vi "Make path.vi"(8 "error in (no error)":errorcluster, 10 "File type":T1, 11 "Tomo in":refnum<class "Tomo.lvclass">) -> (0 "error out":errorcluster, 2 "path":path, 3 "Tomo out":refnum<class "Tomo.lvclass">)   [LabVIEW 2012, in "Tomo.lvclass"]
uses:
  Tomo.lvclass
  file type.ctl
  Tomo.lvclass/Tomo.ctl
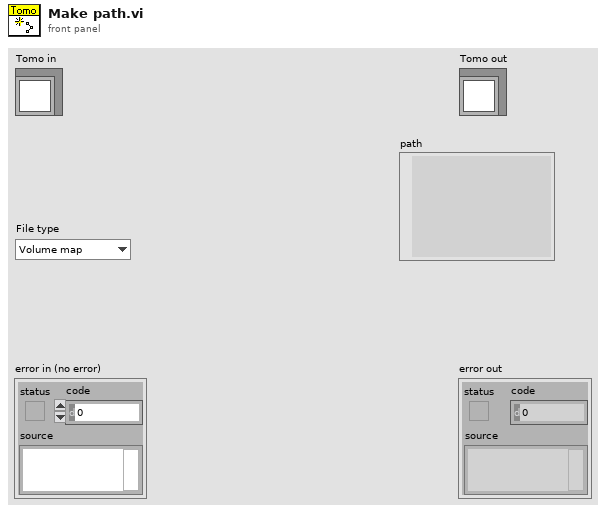
[diagram p1: front panel]
types:
  T1 = typedef "Tomo.lvclass/file type.ctl" = enum16{"Volume map", "Completed stacks"}
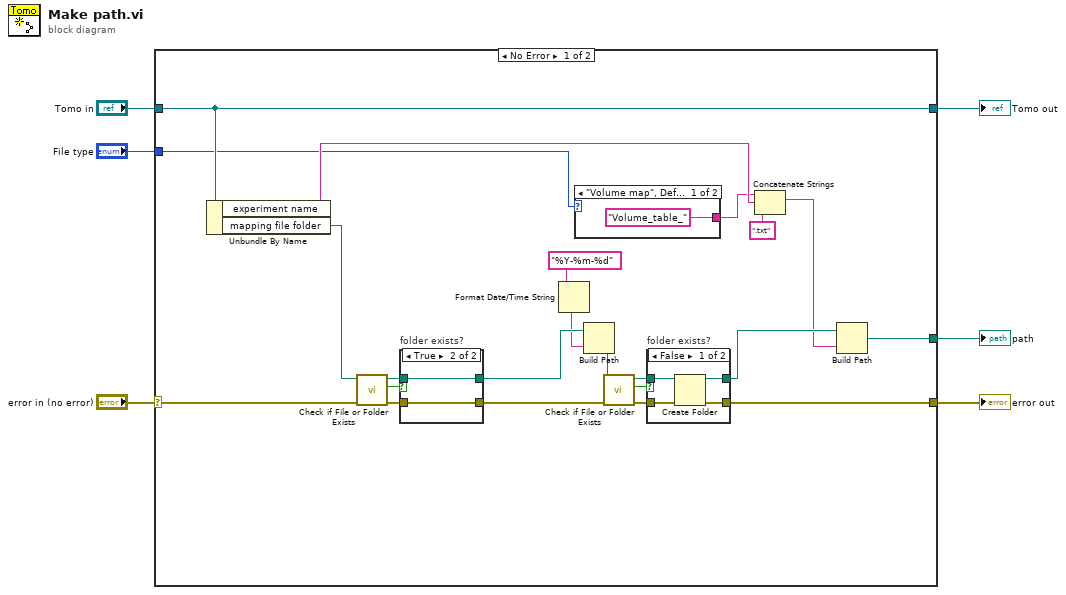
[diagram p0: block diagram]
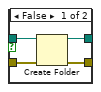
[diagram p3: hidden frame]
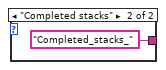
[diagram p4: hidden frame]
diagram:
  n1 = case shown="No Error" "error in (no error)" {
    selector: "error in (no error)" -> [w11 w44]
    tunnel: [w10 w44] -> w5
    tunnel: [w26 w43] -> w3
    tunnel: "Tomo in" -> [w26 w43]
    tunnel: [w7 _] -> w2
    tunnel: "File type" -> [w24 _]
    frame No Error {
      n2 = Unbundle By Name(w26) -> ("experiment name"=w25:string, "mapping file folder"=w22:path)
      n3 = call <vilib>:"Check if File or Folder Exists.vi"("error in (no error)"=w11, "path"=w22) -> ("error out"=w19:errorcluster, "file or folder exists?"=w20:bool, "dup path"=w21:path)  [unwired: 7 in]
      n4 = case "folder exists?" shown="True" w20 {
        tunnel: w21 -> [w38 w40]
        tunnel: w19 -> [w37 w39]
        tunnel: [w36 w39] -> w12
        tunnel: [w35 w40] -> w18
        frame False {
          n5 = Create Folder(path (use dialog)=w38, error in=w37) -> (created path=w35:path, error out=w36:errorcluster)  [unwired: 1 in, 1 out]
        }
        frame True {
        }
      }
      n6 = Format Date/Time String(time format string (%c)="%Y-%m-%d") -> (date/time string=w17:string)  [unwired: 2 out]
      n7 = case shown="\"Volume map\", Default" w24 {
        tunnel: ["Volume_table_" ("string") "Completed_stacks_" ("string")] -> w23
        frame "Volume map", Default {
        }
        frame "Completed stacks" {
        }
      }
      n8 = Build Path(base path=w18, name or relative path=w17) -> (appended path=w13:path)
      n9 = call <vilib>:"Check if File or Folder Exists.vi"("error in (no error)"=w12, "path"=w13) -> ("error out"=w16:errorcluster, "file or folder exists?"=w15:bool, "dup path"=w14:path)  [unwired: 7 in]
      n10 = case "folder exists?" shown="False" w15 {
        tunnel: w14 -> [w32 w34]
        tunnel: w16 -> [w31 w33]
        tunnel: [w30 w33] -> w10
        tunnel: [w29 w34] -> w9
        frame False {
          n11 = Create Folder(path (use dialog)=w32, error in=w31) -> (created path=w29:path, error out=w30:errorcluster)  [unwired: 1 in, 1 out]
        }
        frame True {
        }
      }
      n12 = Concatenate Strings(w23, w25, ".txt" ("string")) -> (w8:string)
      n13 = Build Path(base path=w9, name or relative path=w8) -> (appended path=w7:path)
    }
    frame Error {
    }
  }
  "error out" <- w5
  "Tomo out" <- w3
  "path" <- w2
